vi "String Array to List.vi"(7 "delimiter (, )":string=", ", 10 "string array":string[](array[string])) -> (2 "delimited string":string)   [LabVIEW 2020, in "g-sugar.lvlib"]
doc: "Convert 1D string arrray to a delimited list."
uses:
  g-sugar.lvlib
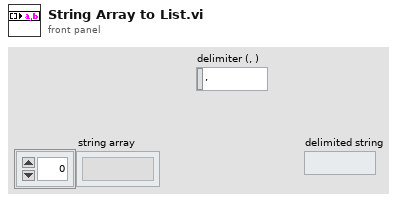
[diagram p1: front panel]
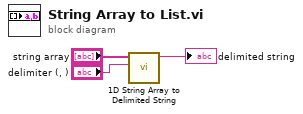
[diagram p0: block diagram]
diagram:
  n1 = call <vilib>:"1D String Array to Delimited String.vi"("delimiter"="delimiter (, )", "string array"="string array") -> ("delimited string"=→"delimited string":string)  [unwired: 9 in]
